vi "iRobot Example - Sensor Stream with Concurrency.vi"() -> ()   [LabVIEW 2013]
doc: "This VI demonstrates how to process sensors in one loop, and simultaneously write commands to the robot in another."
uses:
  Sensor/Sensor Group 6.ctl
  Sensor/Bumps + Wheel Drops.ctl
  Sensor/Low-Side Driver + Wheel Overcurrent.ctl
  Sensor/Buttons.ctl
  Sensor/Charging State.ctl
  Sensor/Cargo Bay Digital Inputs.ctl
  Sensor/Charging Sources Available.ctl
  Sensor/OI Mode.ctl
  Advanced/UART/iRobot UART Port Type.ctl
  Actuator/Drive Direction.ctl
panel:
  in  "UART port":T1
  out "Buttons.Play":bool
  out "Buttons.Advance":bool
  in  "Turn":bool
  in  "Velocity (mm/s)":i16=100
  out "Angle (deg)":i32
  out "Distance (mm)":i32
  out "Bump Right":bool
  out "Bump Left":bool
  in  "Drive":bool
  in  "stop":bool
  out "sensors":T2={"Bumps + Wheel Drops"={"Wheeldrop Caster"=FALSE, "Wheeldrop Left"=FALSE, "Wheeldrop Right"=FALSE, "Bump Left"=FALSE, "Bump Right"=FALSE}, "Wall"=FALSE, "Cliff Left"=FALSE, "Cliff Front Left"=FALSE, "Cliff Front Right"=FALSE, "Cliff Right"=FALSE, "Virtual Wall"=FALSE, "Low-Side Driver + Wheel Overcurrent"={"Low-Side Driver 0"=FALSE, "Low-Side Driver 1"=FALSE, "Low-Side Driver 2"=FALSE, "Left Wheel"=FALSE, "Right Wheel"=FALSE}, "Infrared"=255, "Buttons"={"Advance"=FALSE, "Play"=FALSE}, "Distance (mm)"=0, "Angle (deg)"=0, "Charging State"=enum."Not Charging", "Voltage (mV)"=0, "Current (mA)"=0, "Battery Temperature (deg C)"=0, "Battery Charge (mAh)"=0, "Battery Capacity (mAh)"=0, "Wall Signal (0-4095)"=0, "Cliff Left Signal (0-4095)"=0, "Cliff Front Left Signal (0-4095)"=0, "Cliff Front Right Signal (0-4095)"=0, "Cliff Right Signal (0-4095)"=0, "Cargo Bay Digital Inputs"={"Digital Input 0"=FALSE, "Digital Input 1"=FALSE, "Digital Input 2"=FALSE, "Digital Input 3"=FALSE, "Device Detect"=FALSE}, "Cargo Bay Analog Signal (0-1023)"=0, "Charging Sources Available"={"Internal Charger"=FALSE, "Home Base"=FALSE}, "OI Mode"=enum."Off", "Song Number"=0, "Song Playing"=FALSE, "Number of Stream Packets"=0, "Requested Velocity (mm/s)"=0, "Requested Radius (mm)"=0, "Requested Right Wheel Velocity (mm/s)"=0, "Requested Left Wheel Velocity (mm/s)"=0} {"Infrared" format="%02x"}
  # "Sensors"
  # "Actuators"
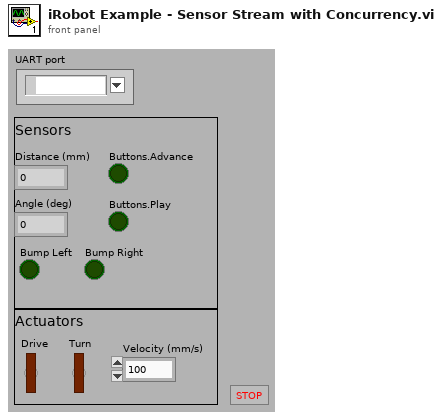
[diagram p1: front panel]
types:
  T1 = typedef "iRobot UART Port Type.ctl" = refnum<visa-resource-name>
  T2 = typedef "Sensor Group 6.ctl" = cluster{"Bumps + Wheel Drops":T3, "Wall":bool, "Cliff Left":bool, "Cliff Front Left":bool, "Cliff Front Right":bool, "Cliff Right":bool, "Virtual Wall":bool, "Low-Side Driver + Wheel Overcurrent":T4, "Infrared":u8, "Buttons":T5, "Distance (mm)":i32, "Angle (deg)":i32, "Charging State":T6, "Voltage (mV)":u16, "Current (mA)":i16, "Battery Temperature (deg C)":i8, "Battery Charge (mAh)":u16, "Battery Capacity (mAh)":u16, "Wall Signal (0-4095)":u16, "Cliff Left Signal (0-4095)":u16, "Cliff Front Left Signal (0-4095)":u16, "Cliff Front Right Signal (0-4095)":u16, "Cliff Right Signal (0-4095)":u16, "Cargo Bay Digital Inputs":T7, "Cargo Bay Analog Signal (0-1023)":u16, "Charging Sources Available":T8, "OI Mode":T9, "Song Number":u8, "Song Playing":bool, "Number of Stream Packets":u8, "Requested Velocity (mm/s)":i16, "Requested Radius (mm)":i16, "Requested Right Wheel Velocity (mm/s)":i16, "Requested Left Wheel Velocity (mm/s)":i16}
  T3 = typedef "Bumps + Wheel Drops.ctl" = cluster{"Wheeldrop Caster":bool, "Wheeldrop Left":bool, "Wheeldrop Right":bool, "Bump Left":bool, "Bump Right":bool}
  T4 = typedef "Low-Side Driver + Wheel Overcurrent.ctl" = cluster{"Low-Side Driver 0":bool, "Low-Side Driver 1":bool, "Low-Side Driver 2":bool, "Left Wheel":bool, "Right Wheel":bool}
  T5 = typedef "Buttons.ctl" = cluster{"Advance":bool, "Play":bool}
  T6 = typedef "Charging State.ctl" = enum16{"Not Charging", "Reconditioning Charging", "Full Charging", "Trickle Charging", "Waiting", "Charging Fault Condition"}
  T7 = typedef "Cargo Bay Digital Inputs.ctl" = cluster{"Digital Input 0":bool, "Digital Input 1":bool, "Digital Input 2":bool, "Digital Input 3":bool, "Device Detect":bool}
  T8 = typedef "Charging Sources Available.ctl" = cluster{"Internal Charger":bool, "Home Base":bool}
  T9 = typedef "OI Mode.ctl" = enum16{"Off", "Passive", "Safe", "Full"}
  T10 = typedef "Drive Direction.ctl" = u16
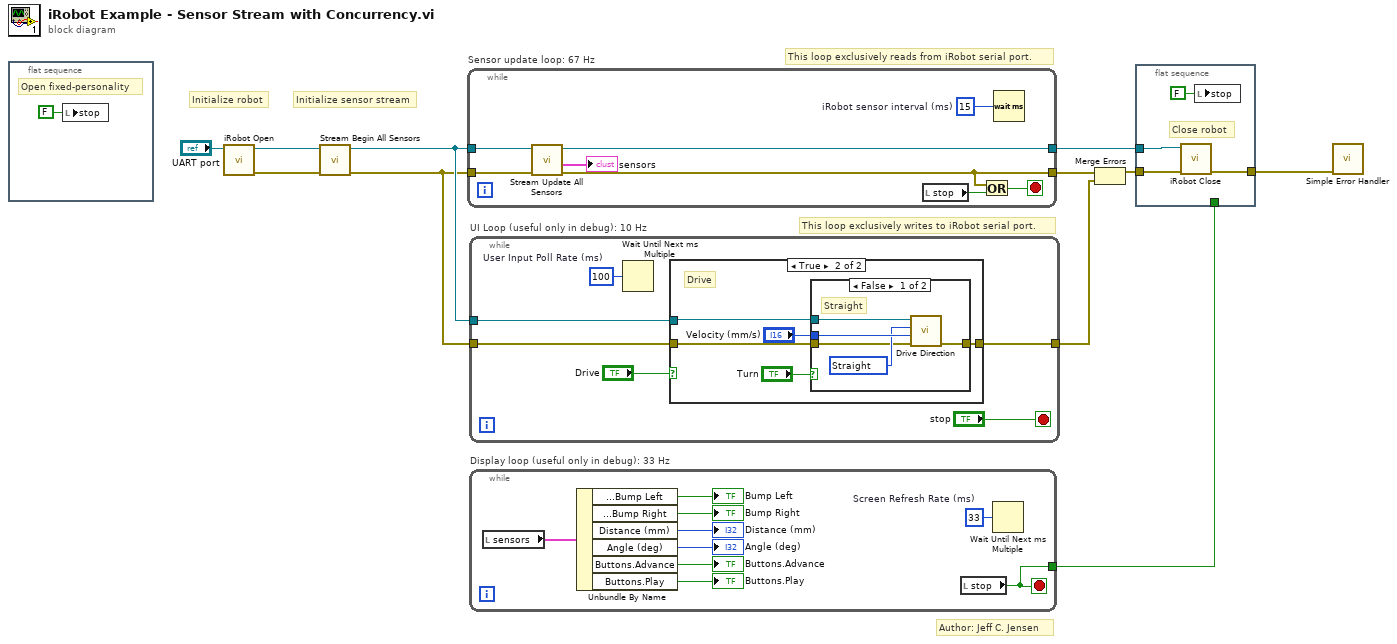
[diagram p0: block diagram]
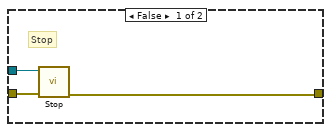
[diagram p2: hidden frame]
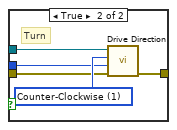
[diagram p3: hidden frame]
diagram:
  # "Initialize sensor stream"
  # "Initialize robot"
  # "This loop exclusively writes to iRobot serial port."
  # "This loop exclusively reads from iRobot serial port."
  # "Author: Jeff C. Jensen"
  n1 = flat-sequence {
    frame #0 {
      # "Open fixed-personality"
      n2 = local write "stop"(FALSE ("stop")) -> ()
    }
  }
  n3 = call "iRobot Open.vi"("UART port in"="UART port") -> ("error out"=w8:errorcluster, "UART port out"=w9:T1)  [unwired: 9 in]
  n4 = call "Stream Begin All Sensors.vi"("error in"=w8, "UART port in"=w9) -> ("error out"=w7:errorcluster, "UART port out"=w10:T1)  [unwired: 8 in]
  n5 = while "Sensor update loop: 67 Hz" {
    tunnel: w10 -> [w20]
    tunnel: [w19] -> w11
    tunnel: w7 -> [w17]
    tunnel: [w13] -> w6
    stop <- w14 stop-if-true
    w16 = u32 15  # iRobot sensor interval (ms)
    n6 = call "Stream Update All Sensors.vi"("error in"=w17, "UART port in"=w20) -> ("error out"=w13:errorcluster, "sensors"=→"sensors":T2, "UART port out"=w19:T1)  [unwired: 5 in, 2 out]
    n7 = local read "stop"() -> (w15:bool)
    n8 = Or(x=w13, y=w15) -> (x .or. y?=w14:bool)
    n9 = Wait (ms)(milliseconds to wait=w16) -> ()  [unwired: 1 out]
  }
  n10 = while "UI Loop (useful only in debug): 10 Hz" {
    tunnel: w10 -> [w24]
    tunnel: w7 -> [w22]
    tunnel: [w21] -> w5
    stop <- "stop" stop-if-true
    w26 = u32 100  # User Input Poll Rate (ms)
    n11 = Wait Until Next ms Multiple(millisecond multiple=w26) -> ()  [unwired: 1 out]
    n12 = case shown="True" "Drive" {
      tunnel: w24 -> [w29 w34]
      tunnel: w22 -> [w28 w31]
      tunnel: [w27 w30] -> w21
      frame False {
        # "Stop"
        n13 = call "Stop.vi"("error in"=w28, "UART port in"=w29) -> ("error out"=w27:errorcluster)  [unwired: 8 in, 1 out]
      }
      frame True {
        # "Drive"
        n14 = case shown="False" "Turn" {
          tunnel: w34 -> [w39 w44]
          tunnel: "Velocity (mm/s)" -> [w38 w42]
          tunnel: w31 -> [w36 w41]
          tunnel: [w35 w40] -> w30
          frame False {
            w37 = T10 32768 items=["Straight"=32768, "Clockwise"=65535, "Counter-Clockwise"=1] ("iRobot Drive Direction")
            # "Straight"
            n15 = call "Drive Direction.vi"("error in"=w36, "Velocity (mm/s)"=w38, "iRobot Drive Direction"=w37, "UART port in"=w39) -> ("error out"=w35:errorcluster)  [unwired: 6 in, 1 out]
          }
          frame True {
            w43 = T10 1 items=["Straight"=32768, "Clockwise"=65535, "Counter-Clockwise"=1] ("iRobot Drive Direction")
            # "Turn"
            n16 = call "Drive Direction.vi"("error in"=w41, "Velocity (mm/s)"=w42, "iRobot Drive Direction"=w43, "UART port in"=w44) -> ("error out"=w40:errorcluster)  [unwired: 6 in, 1 out]
          }
        }
      }
    }
  }
  n17 = while "Display loop (useful only in debug): 33 Hz" {
    tunnel: [w47] -> w3
    stop <- w47 stop-if-true
    w53 = u32 33  # Screen Refresh Rate (ms)
    n18 = local read "sensors"() -> (w52:T2)
    n19 = Unbundle By Name(w52) -> ("Bumps + Wheel Drops.Bump Left"=→"Bump Left":bool, "Bumps + Wheel Drops.Bump Right"=→"Bump Right":bool, "Distance (mm)"=→"Distance (mm)":i32, "Angle (deg)"=→"Angle (deg)":i32, "Buttons.Advance"=→"Buttons.Advance":bool, "Buttons.Play"=→"Buttons.Play":bool)
    n20 = local read "stop"() -> (w47:bool)
    n21 = Wait Until Next ms Multiple(millisecond multiple=w53) -> ()  [unwired: 1 out]
  }
  n22 = Merge Errors(w6, w5) -> (w4:errorcluster)
  n23 = flat-sequence {
    tunnel: w11 -> [w57]
    tunnel: w4 -> [w56]
    tunnel: [w54] -> w2
    tunnel: w3 -> [_]
    frame #0 {
      # "Close robot"
      n24 = call "iRobot Close.vi"("error in"=w56, "UART port in"=w57) -> ("error out"=w54:errorcluster)  [unwired: 9 in]
      n25 = local write "stop"(FALSE ("stop")) -> ()
    }
  }
  n26 = call <vilib>:"Simple Error Handler.vi"("error in (no error)"=w2) -> ()  [unwired: 4 in, 5 out]
